vi "Set Generation Modes.vi"(8 "error in":errorcluster, 10 "DeviceID":T1, 11 "Activation in":refnum<class "Activation.lvclass">) -> (0 "error out":errorcluster, 3 "Activation out":refnum<class "Activation.lvclass">)   [LabVIEW 2018, in "Startup Optimization Actor.lvlib" / "Startup Optimization.lvclass"]
uses:
  Startup Optimization.lvclass
  <vilib>/ORNL/CSEISMIC DDS/CSEISMIC DDS Base/Data Types/Controls/DeviceID.ctl
  Activation Actor/Activation/Activation.lvclass
  C:/Users/Administrator/Desktop/2018LabVIEW EMS/EMS Generic Actor/EMS Generic/EMS Generic.lvclass
  C:/Users/Administrator/Desktop/2018LabVIEW EMS/Device Communication and Control Abstract Actor/Device Communication and Control Abstract/Device Communication and Control Abstract.lvclass
  <vilib>/ORNL/CSEISMIC DDS/CSEISMIC DDS Base/Data Types/DER_setGenerationMode.ctl
  <vilib>/ORNL/CSEISMIC DDS/CSEISMIC DDS Base/Data Types/Controls/Generation Mode.ctl
  <vilib>/ActorFramework/Actor/Actor.lvclass/Actor.ctl
  Device Communication and Control Abstract Actor/Device Communication and Control Abstract/Device Communication and Control Abstract.lvclass/Device Communication and Control Abstract.ctl
  Device Communication and Control Abstract Actor/Device Communication and Control Abstract Messages/Set DER GenerationMode Msg/Set DER GenerationMode Msg.lvclass/Set DER GenerationMode Msg.ctl
  <vilib>/ActorFramework/Message Enqueuer/Message Enqueuer.lvclass/Message Enqueuer.ctl
  Device Communication and Control Abstract Actor/Device Communication and Control Abstract Messages/Set DER GenerationMode Msg/Send Set DER GenerationMode.vi
  <vilib>/ActorFramework/Actor/Read Caller Enqueuer.vi
  <vilib>/ActorFramework/Message Enqueuer/Enqueue.vi
  Device Communication and Control Abstract Actor/Device Communication and Control Abstract/Device Communication and Control Abstract.lvclass
  C:/Program Files (x86)/National Instruments/LabVIEW 2018/vi.lib/ActorFramework/Actor/Actor.lvclass
  Device Communication and Control Abstract Actor/Device Communication and Control Abstract Messages/Set DER GenerationMode Msg/Set DER GenerationMode Msg.lvclass
  C:/Program Files (x86)/National Instruments/LabVIEW 2018/vi.lib/ActorFramework/Message/Message.lvclass
  <vilib>/ActorFramework/Message Priority Queue/Priority Enqueue.vi
  <vilib>/ORNL/CSEISMIC DDS/CSEISMIC DDS Base/CSEISMIC DDS.lvclass
  EMS Generic Actor/EMS Generic/EMS Generic.lvclass
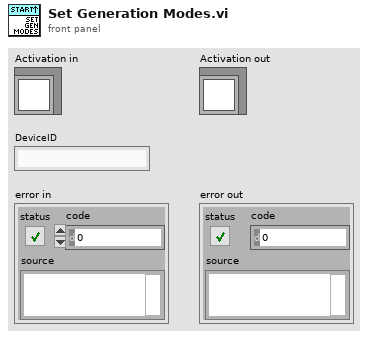
[diagram p1: front panel]
types:
  T1 = typedef "CSEISMIC DDS.lvlib/CSEISMIC DDS.lvclass/DeviceID.ctl" = string
  T2 = typedef "CSEISMIC DDS.lvlib/CSEISMIC DDS.lvclass/IED_Status.ctl" = cluster{"DeviceID":T1, "Timestamp":T3, "MicrogridID":u8, "Active":bool, "Inactive":bool, "Error":i32, "Fault":bool, "ErrorString":string}
  T3 = typedef "CSEISMIC DDS.lvlib/CSEISMIC DDS.lvclass/Timestamp.ctl" = cluster{"Seconds":u64, "Remainder":u64}
  T4 = typedef "CSEISMIC DDS.lvlib/CSEISMIC DDS.lvclass/DER_setGenerationMode.ctl" = cluster{"DeviceID":T1, "Mode":T5}
  T5 = typedef "CSEISMIC DDS.lvlib/CSEISMIC DDS.lvclass/Generation Mode.ctl" = enum32{"Invalid", "PQ", "Droop", "PV", "PF", "VF"}
  T6 = typedef "CSEISMIC DDS.lvlib/CSEISMIC DDS.lvclass/DER_Status.ctl" = cluster{"DeviceID":T1, "VFControl":bool, "PControl":bool, "QControl":bool, "PFControl":bool, "PVControl":bool, "Droop":bool, "Unbalanced":bool, "MicrogridVF":bool, "RealDroop(kW)":T7, "ReactiveDroop(kVar)":T7}
  T7 = typedef "CSEISMIC DDS.lvlib/CSEISMIC DDS.lvclass/DroopCurve.ctl" = cluster{"XMin":dbl, "XMax":dbl, "YMin":dbl, "YMax":dbl}
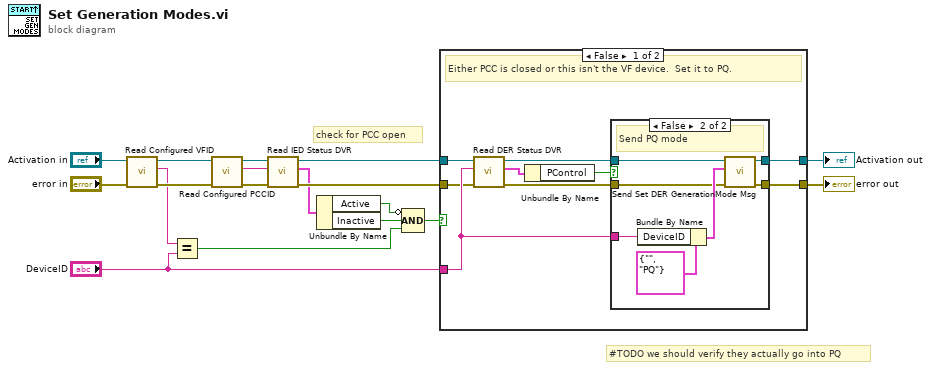
[diagram p0: block diagram]
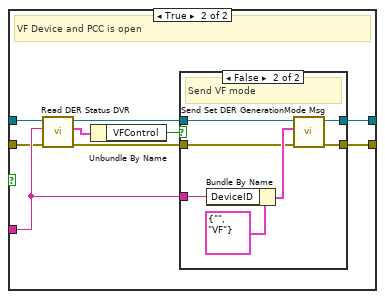
[diagram p3: hidden frame]
diagram:
  # "#TODO we should verify they actually go into PQ"
  # "check for PCC open"
  n1 = call "Read Configured VFID.vi"("error in"="error in", "EMS Generic in"="Activation in") -> ("error out"=w13:errorcluster, "VFID"=w12:T1, "EMS Generic out"=w15:refnum<class "Activation.lvclass">)  [unwired: 7 in]
  n2 = Equal?(x=w12, y="DeviceID") -> (x = y?=w2:bool)
  n3 = call "Read Configured PCCID.vi"("error in"=w13, "EMS Generic in"=w15) -> ("error out"=w9:errorcluster, "PCCID"=w6:T1, "EMS Generic out"=w10:refnum<class "Activation.lvclass">)  [unwired: 7 in]
  n4 = call "Read IED Status DVR.vi"("error in"=w9, "DeviceID"=w6, "EMS Generic in"=w10) -> ("error out"=w8:errorcluster, "IED_Status"=w5:T2, "EMS Generic out"=w7:refnum<class "Activation.lvclass">)  [unwired: 5 in, 1 out]
  n5 = Unbundle By Name(w5) -> ("Active"=w4:bool, "Inactive"=w3:bool)
  n6 = Compound Arithmetic op=AND(invert w4, w3, w2) -> (w1:bool)
  n7 = case shown="False" w1 {
    tunnel: [w27 w45] -> w18
    tunnel: [w26 w44] -> w17
    tunnel: "DeviceID" -> [w25 w43]
    tunnel: w8 -> [w20 w38]
    tunnel: w7 -> [w19 w37]
    frame False {
      # "Either PCC is closed or this isn't the VF device.  Set it to PQ."
      n8 = call "Read DER Status DVR.vi"("error in"=w20, "DeviceID"=w25, "EMS Generic in"=w19) -> ("error out"=w22:errorcluster, "DER_Status"=w23:T6, "EMS Generic out"=w21:refnum<class "Activation.lvclass">)  [unwired: 5 in, 1 out]
      n9 = Unbundle By Name(w23) -> ("PControl"=w24:bool)
      n10 = case shown="False" w24 {
        tunnel: w22 -> [w29 w34]
        tunnel: w21 -> [w28 w33]
        tunnel: [w28 w32] -> w26
        tunnel: [w29 w31] -> w27
        tunnel: w25 -> [_ w30]
        frame True {
          # "Already in PQ. Do nothing."
        }
        frame False {
          # "Send PQ mode"
          n11 = Bundle By Name(cluster=T4 {"DeviceID"="", "Mode"=enum."PQ"} ("DER_setGenerationMode"), "DeviceID"=w30) -> (w36:T4)
          n12 = call "Send Set DER GenerationMode Msg.vi"("error in"=w34, "DER_setGenerationMode"=w36, "SCADA Sub Abstract in"=w33) -> ("error out"=w31:errorcluster, "SCADA Sub Abstract out"=w32:refnum<class "Activation.lvclass">)  [unwired: 7 in]
        }
      }
    }
    frame True {
      # "VF Device and PCC is open"
      n13 = call "Read DER Status DVR.vi"("error in"=w38, "DeviceID"=w43, "EMS Generic in"=w37) -> ("error out"=w40:errorcluster, "DER_Status"=w41:T6, "EMS Generic out"=w39:refnum<class "Activation.lvclass">)  [unwired: 5 in, 1 out]
      n14 = Unbundle By Name(w41) -> ("VFControl"=w42:bool)
      n15 = case shown="False" w42 {
        tunnel: w40 -> [w47 w52]
        tunnel: w39 -> [w46 w51]
        tunnel: [w46 w50] -> w44
        tunnel: [w47 w49] -> w45
        tunnel: w43 -> [_ w48]
        frame True {
          # "Already in VF. Do nothing."
        }
        frame False {
          # "Send VF mode"
          n16 = Bundle By Name(cluster=T4 {"DeviceID"="", "Mode"=enum."VF"} ("DER_setGenerationMode"), "DeviceID"=w48) -> (w54:T4)
          n17 = call "Send Set DER GenerationMode Msg.vi"("error in"=w52, "DER_setGenerationMode"=w54, "SCADA Sub Abstract in"=w51) -> ("error out"=w49:errorcluster, "SCADA Sub Abstract out"=w50:refnum<class "Activation.lvclass">)  [unwired: 7 in]
        }
      }
    }
  }
  "error out" <- w18
  "Activation out" <- w17
